vi "Remove Semicolon.vi"(11 "String In":string) -> (3 "String Out":string)   [LabVIEW 2021]
doc: "delete semicolon from input string"
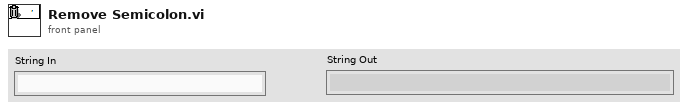
[diagram p1: front panel]
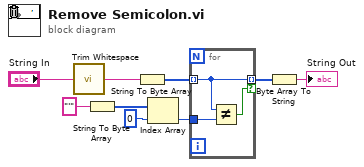
[diagram p0: block diagram]
diagram:
  n1 = call <vilib>:"Trim Whitespace.vi"("string"="String In") -> ("trimmed string"=w8:string)  [unwired: 1 in]
  n2 = String To Byte Array(string="'") -> (unsigned byte array=w5:u8[])
  n3 = String To Byte Array(string=w8) -> (unsigned byte array=w6:u8[])
  n4 = Index Array(array=w5, index=0) -> (element=w4:u8)
  n5 = for {
    tunnel: w6 -> [w11] mode=indexing
    tunnel: w4 -> [w12]
    tunnel: [w11] -> w2 mode=indexing if=w10
    n6 = Not Equal?(x=w11, y=w12) -> (x != y?=w10:bool)
  }
  n7 = Byte Array To String(unsigned byte array=w2) -> (string=→"String Out":string)
